vi "ATF-P&ID.vi"() -> ()   [LabVIEW 2022 SP3]
uses:
  Source code/Globals/Main_global.vi
  Source code/Globals/ATF1_NS_globals.vi
  <vilib>/Utility/error.llb/DialogType.ctl
  <vilib>/Waveform/DWDTOps.llb/DWDT Digital to Boolean Array.vi
  Source code/Globals/ATF1_ACQ.vi
  Source code/ATF_Queues/ATF_Message Cluster.ctl
  Source code/User Event - Stop/User Event - Stop.lvlib
  <vilib>/Analysis/3filter.llb/Filter Passband Type.ctl
  <vilib>/Analysis/NI_AALBase.lvlib
  <vilib>/ptbypt/NI_PtbyPt.lvlib
panel:
  out "Boolean 73":bool
  out "Boolean 30":bool
  in  "F EPV 1008":bool
  out "NC EPV 1008 HSS":bool
  out "Boolean 27":bool
  in  "F EPV 1007":bool
  out "F EPV 1007 HSS":bool
  in  "F EPV 1004":bool
  out "NC EPV 1004 HSS":bool
  out "Boolean 26":bool
  in  "NC EPV 1001":bool
  out "NC EPV 1001 HSS":bool
  out "Boolean 23":bool
  out "Boolean 25":bool
  out "NO EPV 477 HSS  3":bool
  in  "NC EPV 61":bool
  out "Boolean 104":bool
  out "Boolean 47":bool
  out "Boolean 3":bool
  out "Boolean 24":bool
  out "NC EPV 56 HSS":bool
  in  "NC EPV 56":bool
  out "Boolean 16":bool
  out "Boolean 116":bool
  in  "NO EPV 122":bool
  out "Boolean 46":bool
  out "NO EPV 1102 HSS 2":bool
  out "Boolean 103":bool
  out "F_RTD_56(K)":dbl format="%.2g"
  out "N_PT_121":dbl format="%.2g"
  out "WTT_LS 2":dbl(slide) scale=0.1..100.0
  out "Boolean 71":bool
  out "F_RTD_1013 (K)":dbl format="%.2g"
  out "PT SC":dbl format="%.2g"
  out "W_RTD_1177 (K)":dbl format="%.2g"
  out "F_SC_RTD(K)":dbl format="%.2g"
  out "PT 1000(K)":dbl format="%.2g"
  out "PT 1000-2 (K)":dbl format="%.2g"
  out "F_PT_1013b (bar)":dbl format="%.2g"
  out "F_PT_1013a (bar)":dbl format="%.2g"
  out "F_PT_1019":dbl format="%.2g"
  out "F_TCV_1018":dbl format="%.2g"
  out "TCV_1018(FB) %":dbl format="%.2g"
  out "Boolean 108":bool
  out "Boolean 107":bool
  out "F_RTD_1011(K)":dbl format="%.2g"
  out "Boolean 21":bool
  out "Boolean 138":bool
  out "Boolean 29":bool
  out "Boolean 28":bool
  out "F_PT_1011a (bar)":dbl format="%.2g"
  out "F_PT_1011b (bar)":dbl format="%.2g"
  out "F_FM_1010 (kg/s)":dbl format="%.2g"
  out "Boolean 106":bool
  out "Boolean 105":bool
  out "Boolean 121":bool
  out "Boolean 126":bool
  out "Boolean 109":bool
  out "Boolean 6":bool
  out "Boolean 81":bool
  out "NO EPV 477 HSS  2":bool
  in  "NO EPV 477":bool
  in  "NO EPV 478R":bool
  out "NO EPV 1207 HSS 2":bool
  out "Boolean 54":bool
  out "Boolean 53":bool
  out "Boolean 22":bool
  out "Boolean 86":bool
  out "F_PT_56 _R":dbl format="%.2g"
  in  "NC EPV 481":bool
  out "NC EPV 481 HSS":bool
  out "Boolean 85":bool
  out "F_PT_56":dbl format="%.2g"
  out "Boolean 115":bool
  out "Boolean 52":bool
  out "N_PT_480":dbl format="%.2g"
  out "Boolean 120":bool
  out "Boolean 72":bool
  out "Boolean 119":bool
  out "Boolean 13":bool
  out "N_PT_ATF_Cyl":dbl format="%.2g"
  out "Boolean 83":bool
  out "Boolean 102":bool
  out "Boolean 82":bool
  out "Boolean 101":bool
  out "N_PT_1101":dbl format="%.2g"
  out "N_PT_1090   2":dbl format="%.2g"
  in  "N EPV 1091":bool
  out "NO EPV 1091 HSS":bool
  out "Boolean 20":bool
  out "Boolean 118":bool
  in  "NC EPV 1217":bool
  out "NC EPV 1217 HSS":bool
  out "Boolean 4":bool
  out "Boolean 114":bool
  out "Boolean 12":bool
  out "N_PT_Water_Cyl":dbl format="%.2g"
  out "Boolean 79":bool
  out "N_PT_1210":dbl format="%.2g"
  out "Boolean 117":bool
  out "W_PT_1212":dbl format="%.2g"
  out "W_RTD_1212(K)":dbl format="%.2g"
  out "Boolean 19":bool
  out "Boolean 18":bool
  out "Boolean 8":bool
  out "Boolean 15":bool
  out "Boolean 14":bool
  out "Boolean 11":bool
  out "Boolean 10":bool
  in  "AC Button":bool
  in  "NO EPV 1207":bool
  out "Boolean 7":bool
  out "Boolean 5":bool
  in  "NC EPV 1214":bool
  out "Boolean 141":bool
  out "Boolean 9":bool
  out "WTT_LS":dbl(slide) scale=0.1..100.0
  out "Boolean 140":bool
  out "Boolean 144":bool
  out "Boolean 128":bool
  out "Boolean 125":bool
  in  "NO EPV 1102":bool
  out "Boolean 45":bool
  out "NC EPV 1211 HSS":bool
  in  "NC EPV 1211":bool
  out "NO EPV 1207 HSS":bool
  out "NC EPV 1214 HSS":bool
  out "NO EPV 1102 HSS":bool
  out "Boolean 113":bool
  out "Boolean 2":bool
  out "Boolean 100":bool
  out "Boolean 80":bool
  out "Boolean 78":bool
  out "Boolean 70":bool
  out "Boolean":bool
  out "Boolean 51":bool
  out "Boolean 17":bool
  out "Boolean 112":bool
  out "error out":errorcluster
  out "Sampling Rate_Accelerometer":dbl
  out "register values":u16[](array[numeric])
  # "ATF PUMP & STOORAGE P&ID"
  # "WTT\nh(mm)"
  # "ATF"
  # "ATF"
  # "ATF STORAGE\nAREA"
  # "ATF PUMP\nAREA"
  # "GN2"
  # "GN2"
  # "Version:V0.1"
  # "Release Date:14/10/2024"
  # "GN2"
  # "GN2"
  # "GN2"
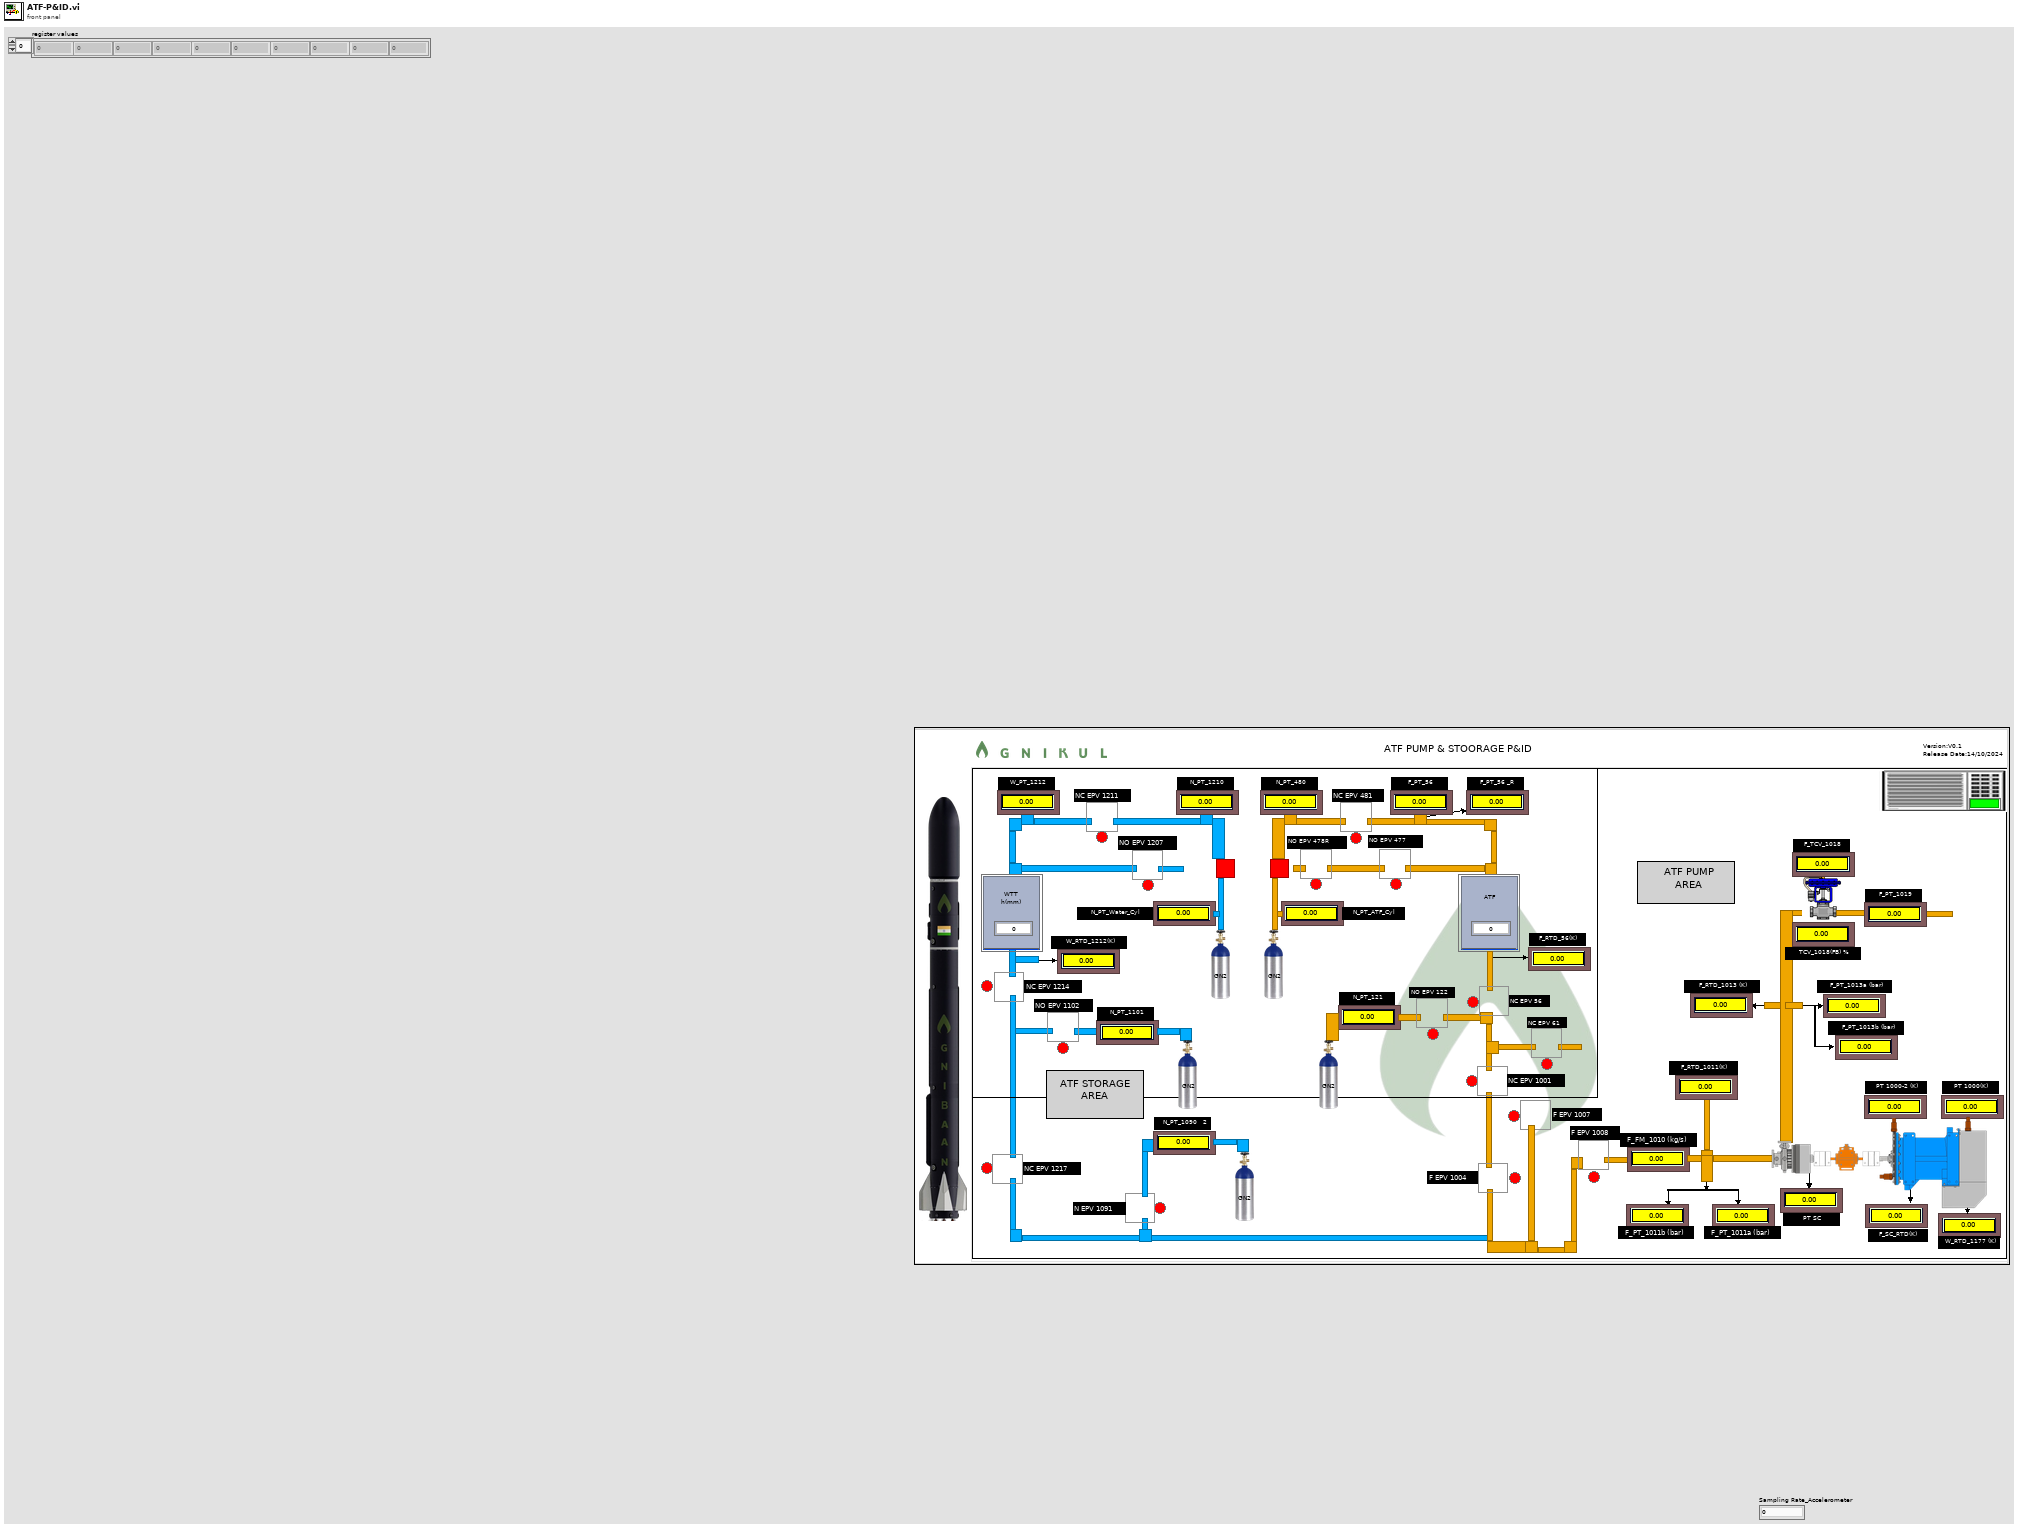
[diagram p1: front panel]
types:
  T1 = cluster{"DO Data":waveform(dbl)[], "DI Data":digitalwaveform[], "AI Data":waveform(dbl)[]}
  T2 = enum8{"Enabled", "Disabled", "Disabled and Grayed Out"}
  T3 = cluster{"UI":refnum<queue>, "Acquisition":refnum<queue>, "Logging":refnum<queue>}
  T4 = cluster{cluster{"AI":cluster{"AI signal Lists":string, "AI Channel List":string, "Prescale Min":dbl, "Prescale Max":dbl, "Prescale Unit":string, "Sensor Min":dbl, "Sensor Max":dbl, "Sensor Unit":string}[], "AI Sample rate":u32[], "AI Device list ":string[]}, cluster{"AO":cluster{"AO signal List":string, "AO Channel List":string, "AO Default Value":dbl}[], "AO Sample rate ":u32[], "AO Device list":string[]}, cluster{"DI":cluster{"DI Signal List":string, "DI Channel list":string, "Default":bool, "Inverted":bool}[], "DI Sample rate":u32[], "DI Device list  ":string[]}, cluster{"DO":cluster{"DO Signal List":string, "DO Channel List":string, "DO Default":bool, "DO Inverted":bool}[], "DO Sample rate":u32[], "DO Device list ":string[]}, cluster{"CI":cluster{"CI Signal list":string, "CI Channel List":string, "Initial Count":u32, "Count Direction":i32, "Edge":i32}[], "CI Sample rate":u32[], "CI Device list ":string[]}, cluster{"TC":cluster{"TC signal Lists":string, "TC Channel Lists":string, "TC type":i32, "Max.Value":dbl, "Min.Value":dbl, "Units":i32}[], "TC Sample rate":u32[], "TC Device list":string[]}, cluster{"Accelerometer":cluster{"name to assign":string, "physical channels":tag, "minimum value":dbl, "maximum value":dbl, "sensitivity":dbl, "sensitivity units":i32, "units":i32}[], "Acc Sampling Rate":string}}
  T5 = enum32{"Invalid", "Standard", "Closed", "Hidden", "Minimized", "Maximized"}
  T6 = typedef "Control 3.ctl" = cluster{"Info  Folder path":path, " Data Log Folder Path ":path, " Error log Folder Path":path, "Login Details  Folder Path":path, "HW Configaration  Folder Path":path, "Signal Folder Path":path, "Test Settings Data Log Folder Path ":path, "System Setting Sequence Folder Path":path, "Sequence Folder Path":path, "Sub VI's  Folder Path":path, "DAQ  VI's  Folder Path":path, "Source Code  Folder Path":path, "Log In Module  Folder Path ":path, "Button Operations Folder Path":path, "Loading Vi path":path, "Loading Vi path D":path}
  T7 = typedef "ATF_Message Cluster.ctl" = cluster{"Message":string, "Message Data":variant}
  T8 = typedef "DialogType.ctl" = u16
  T9 = typedef "NI_AALBase.lvlib/Filter Passband Type.ctl" = enum32{"Lowpass", "Highpass", "Bandpass", "Bandstop"}
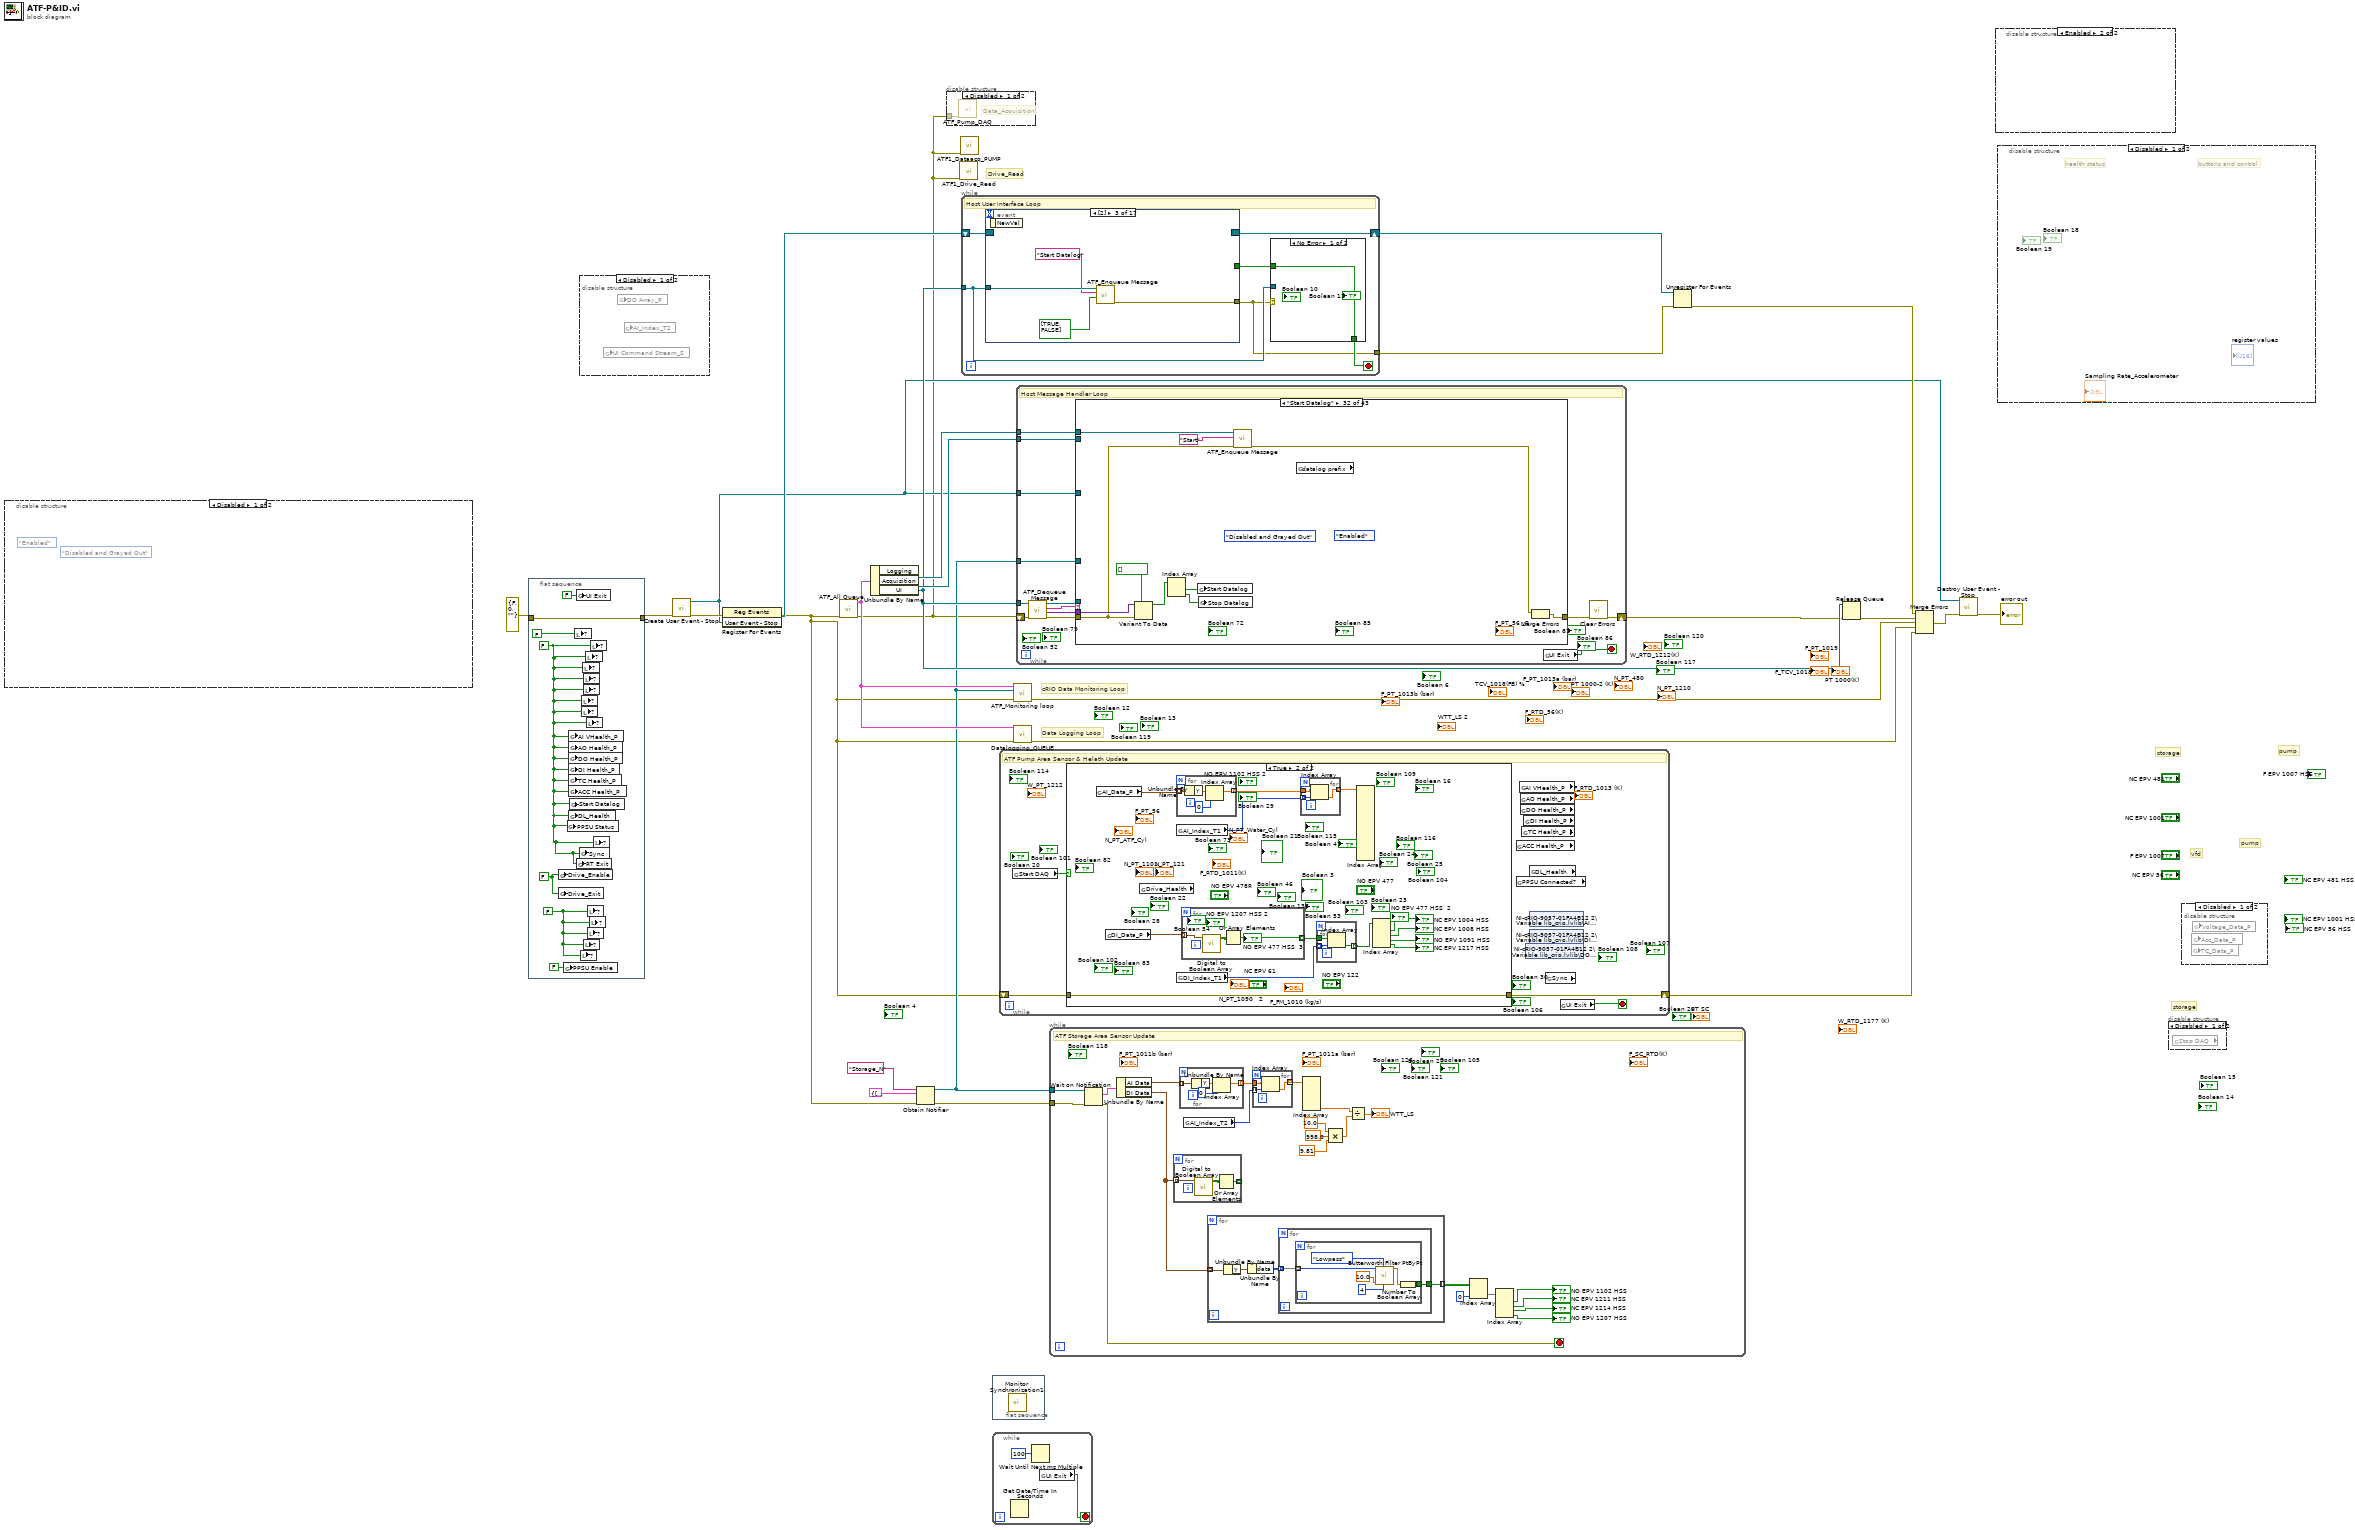
[diagram p0: block diagram]
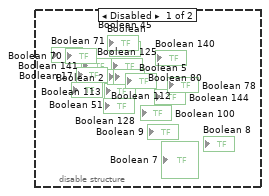
[diagram p7: hidden frame]
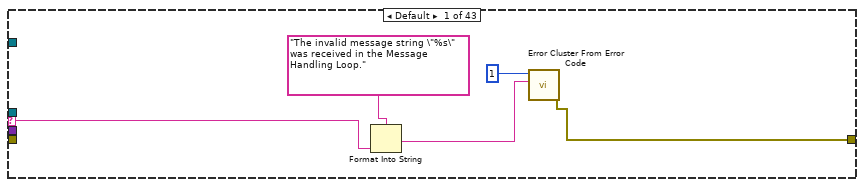
[diagram p9: hidden frame]
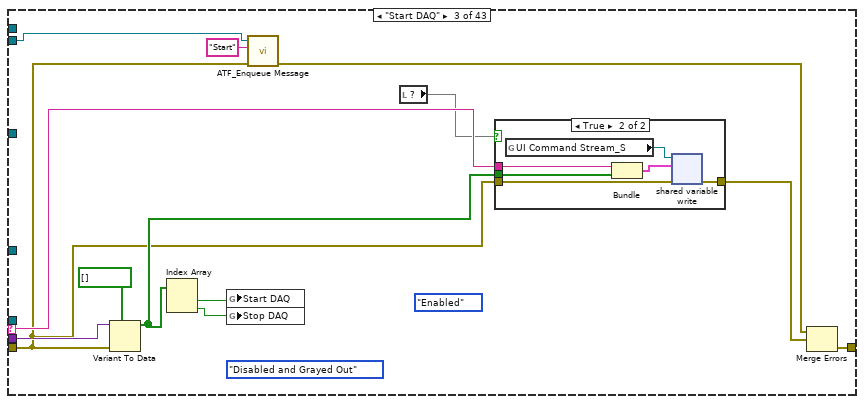
[diagram p11: hidden frame]
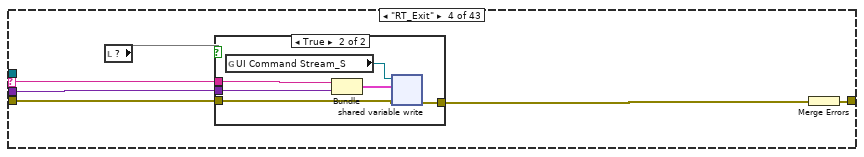
[diagram p13: hidden frame]
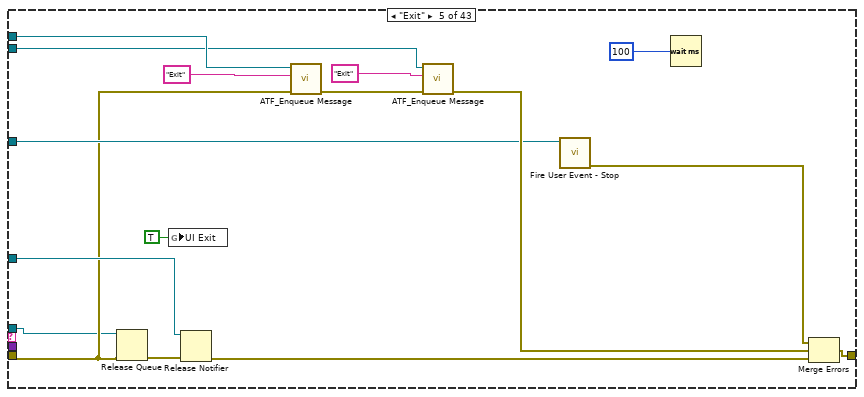
[diagram p15: hidden frame]
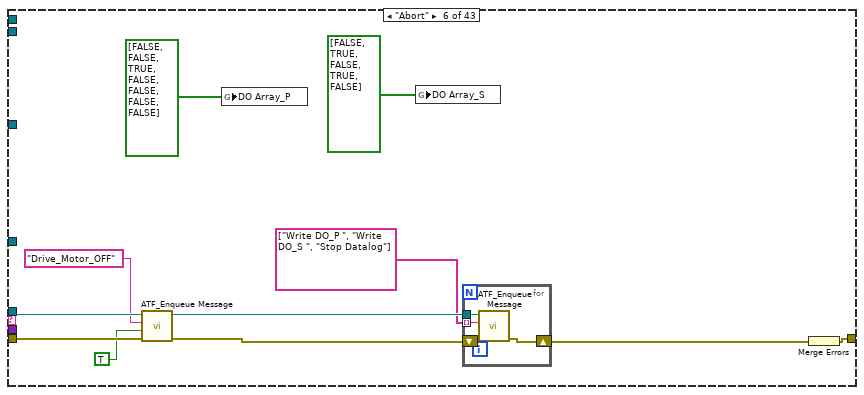
[diagram p16: hidden frame]
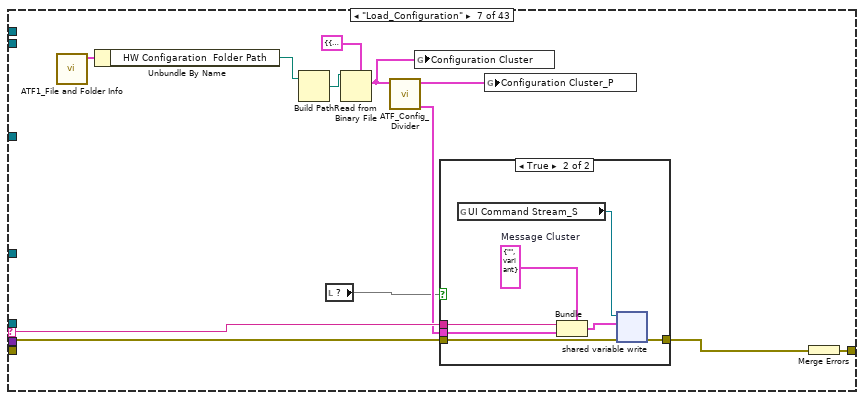
[diagram p17: hidden frame]
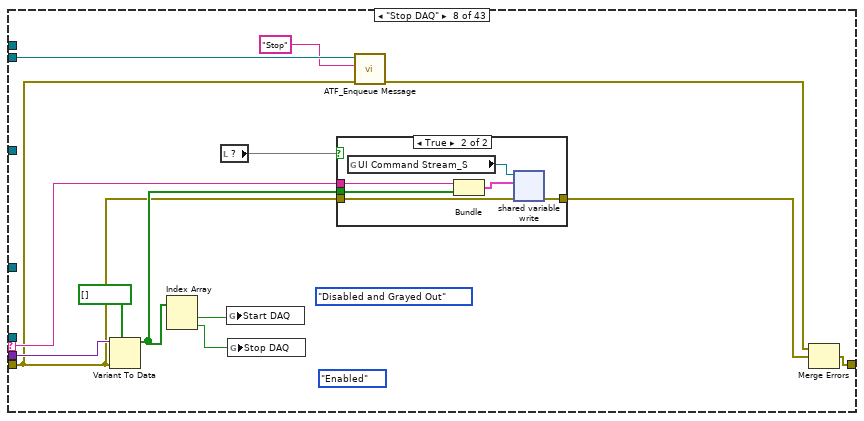
[diagram p19: hidden frame]
diagram:
  # "Data Logging Loop"
  # "cRIO Data Monitoring Loop"
  # "Drive_Read"
  # "pump"
  # "vfd"
  # "pump"
  # "storage"
  # "storage"
  n1 = disable-structure shown="Disabled" {
    frame Disabled {
      w27 = T2."Disabled and Grayed Out" ("Disabled")
      w26 = T2."Enabled" ("Disabled")
    }
    frame Enabled {
    }
  }
  n2 = flat-sequence {
    tunnel: [w29] -> w4
    tunnel: errorcluster {"status"=FALSE, "code"=0, "source"=""} ("error in (no error)") -> [w29]
    frame #0 {
      w31 = FALSE ("DI Health cRIO")
      w32 = FALSE ("Drive Connected?")
      w28 = FALSE ("Datalog Health")
      n3 = global write "ATF1_ACQ.vi" "Drive_Enable"(w32) -> ()
      n4 = global write "ATF1_ACQ.vi" "Drive_Exit"(w32) -> ()
      n5 = global write "Main_global.vi" "PPSU Enable"(FALSE ("PPSU Enable")) -> ()
      n6 = global write "ATF1_ACQ.vi" "PPSU Status"(w28) -> ()
      n7 = global write "ATF1_ACQ.vi" "AI VHealth_P"(w28) -> ()
      n8 = global write "ATF1_ACQ.vi" "AO Health_P"(w28) -> ()
      n9 = global write "ATF1_ACQ.vi" "DO Health_P"(w28) -> ()
      n10 = global write "ATF1_ACQ.vi" "DI Health_P"(w28) -> ()
      n11 = global write "ATF1_ACQ.vi" "TC Health_P"(w28) -> ()
      n12 = global write "ATF1_ACQ.vi" "ACC Health_P"(w28) -> ()
      n13 = global write "Main_global.vi" "DL_Health"(w28) -> ()
      n14 = global write "Main_global.vi" "Start Datalog"(w28) -> ()
      n15 = local write item#-1(FALSE ("PUMP Connected?")) -> ()
      n16 = global write "Main_global.vi" "UI Exit"(FALSE ("UI Exit")) -> ()
      n17 = global write "Main_global.vi" "RT Exit"(w28) -> ()
      n18 = global write "Main_global.vi" "Sync"(w28) -> ()
      n19 = local write item#-1(w31) -> ()
      n20 = local write item#-1(w28) -> ()
      n21 = local write item#-1(w28) -> ()
      n22 = local write item#-1(w28) -> ()
      n23 = local write item#-1(w28) -> ()
      n24 = local write item#-1(w28) -> ()
      n25 = local write item#-1(w31) -> ()
      n26 = local write item#-1(w28) -> ()
      n27 = local write item#-1(w28) -> ()
      n28 = local write item#-1(w31) -> ()
      n29 = local write item#-1(w31) -> ()
      n30 = local write item#-1(w31) -> ()
      n31 = local write item#-1(w28) -> ()
      n32 = local write item#-1(w28) -> ()
    }
  }
  n33 = disable-structure shown="Disabled" {
    frame Disabled {
      n34 = global read "ATF1_NS_globals.vi" "UI Command Stream_S"() -> ()  [unwired: 1 in]
      n35 = global read "ATF1_ACQ.vi" "DO Array_P"() -> ()  [unwired: 1 in]
      n36 = global read "Main_global.vi" "AI_Index_T2"() -> ()  [unwired: 1 in]
    }
    frame Enabled {
    }
  }
  n37 = call "Create User Event - Stop.vi"("error in (no error)"=w4) -> ("error out"=w13:errorcluster, "User Event - Stop"=w6:refnum<user-event>)  [unwired: 9 in]
  n38 = register-events(error in=w13, w6) -> (reference out=w12:refnum<event-registration>, error out=w2:errorcluster)  [unwired: 1 in]
  n39 = call "ATF_All Queue.vi"("error in"=w2) -> ("error out"=w1:errorcluster, "Cluster"=w19:T3)  [unwired: 9 in]
  n40 = Unbundle By Name(w19) -> ("Logging"=w25:refnum<queue>, "Acquisition"=w24:refnum<queue>, "UI"=w23:refnum<queue>)
  n41 = Obtain Notifier(name (unnamed)="Storage_N", notification data type=T1 {"DO Data"=[], "DI Data"=[], "AI Data"=[]}, error in (no error)=w2) -> (notifier out=w14:refnum<notifier>, error out=w16:errorcluster)  [unwired: 1 in, 1 out]
  n42 = disable-structure shown="Disabled" {
    disable-tunnel: w1 -> [w35 _]
    frame Disabled {
      # "Data_Acquisition"
      n43 = call "ATF_Pump_DAQ.vi"("error constant"=w35) -> ()  [unwired: 10 in, 1 out]
    }
    frame Enabled {
    }
  }
  n44 = call "ATF1_Drive_Read.vi"("error in (no error)"=w1) -> ()  [unwired: 10 in, 1 out]
  n45 = call "ATF1_Dataacq_PUMP.vi"("error In"=w1) -> ()  [unwired: 10 in, 1 out]
  n46 = while {
    tunnel: w23 -> [w41]
    shift-right: [w37] -> w10
    shift-left: w12 -> [w38]
    tunnel: [w36] -> w11
    stop <- w40 stop-if-true
    # "Host User Interface Loop"
    n47 = event shown="[2]" {
      selector: w38 -> [_ _ _ _ _ _ _ _ _ _ _ _ _ _ _ _ _]
      dyn-events: [_ _ _ _ _ _ _ _ _ _ _ _ _ _ _ _ _] -> w37
      timeout: _ -> [_ _ _ _ _ _ _ _ _ _ _ _ _ _ _ _ _]
      tunnel: w41 -> [w49 w61 w65 w68 w72 w77 w82 w86 w90 w94 w97 w101 w105 w108 w111 _ w118]
      tunnel: [w53 w60 w64 w67 w71 w76 w81 w85 w89 w93 w96 w100 w104 w107 w110 _ w116] -> w36
      tunnel: [_ _ _ _ _ TRUE _ _ _ _ _ _ _ _ _ TRUE ("Discard?") _] -> w39
      event #0 (no event record) {
        n48 = event-data() -> ()  [unwired: 1 in, 1 out]
        n49 = for {
          tunnel: [w57] -> w50
          tunnel: w49 -> [w56]
          tunnel: [w55] -> w48
          tunnel: string[] ["Load_Configuration", "Signal_List", "Indexing", "Update DO_P", "Update DO_S", "Write DO_P", "Write DO_S"] -> [w54] mode=indexing
          n50 = call "ATF_Enqueue Message.vi"("Message"=w54, "Message Queue"=w56) -> ("error out"=w57:errorcluster, "dup Message Queue"=w55:refnum<queue>)  [unwired: 8 in]
        }
        n51 = call "ATF_Enqueue Message.vi"("error in (no error)"=w50, "Message Data"=bool[] [TRUE, FALSE], "Message"="Start DAQ", "Message Queue"=w48) -> ("error out"=w53:errorcluster)  [unwired: 6 in, 1 out]
      }
      event #1 (no event record) {
        n52 = event-data() -> ()  [unwired: 1 in, 1 out]
        n53 = call "ATF_Enqueue Message.vi"("Message Data"=bool[] [FALSE, TRUE], "Message"="Stop DAQ", "Message Queue"=w61) -> ("error out"=w60:errorcluster)  [unwired: 7 in, 1 out]
      }
      event #2 (no event record) {
        n54 = event-data() -> ()  [unwired: 1 in, 1 out]
        n55 = call "ATF_Enqueue Message.vi"("Message Data"=bool[] [TRUE, FALSE], "Message"="Start Datalog", "Message Queue"=w65) -> ("error out"=w64:errorcluster)  [unwired: 7 in, 1 out]
      }
      event #3 (no event record) {
        n56 = event-data() -> ()  [unwired: 1 in, 1 out]
        n57 = call "ATF_Enqueue Message.vi"("Message"="Rename_Datalog", "Message Queue"=w68) -> ("error out"=w67:errorcluster)  [unwired: 8 in, 1 out]
      }
      event #4 (no event record) {
        n58 = event-data() -> ()  [unwired: 1 in, 1 out]
        n59 = call "ATF_Enqueue Message.vi"("Message Data"=bool[] [FALSE, TRUE], "Message"="Stop Datalog", "Message Queue"=w72) -> ("error out"=w71:errorcluster)  [unwired: 7 in, 1 out]
      }
      event #5 (no event record) {
        n60 = event-data() -> ()  [unwired: 1 in, 1 out]
        n61 = call "ATF_Enqueue Message.vi"("Message"="Exit", "Message Queue"=w77) -> ("error out"=w76:errorcluster, "Message Data"=w73:variant)  [unwired: 7 in, 1 out]
      }
      event #6 (no event record) {
        n62 = event-data() -> ("NewVal"=w79)  [unwired: 1 in]
        n63 = call "ATF_Enqueue Message.vi"("Message Data"=w79, "Message"="RT_Exit", "Message Queue"=w82) -> ("error out"=w81:errorcluster)  [unwired: 7 in, 1 out]
        n64 = global read "Main_global.vi" "RT Exit"() -> (w78:bool)
      }
      event #7 (no event record) {
        n65 = event-data() -> ("NewVal"=w83)  [unwired: 1 in]
        n66 = call "ATF_Enqueue Message.vi"("Message Data"=w83, "Message"="DAQ_Configuration", "Message Queue"=w86) -> ("error out"=w85:errorcluster)  [unwired: 7 in, 1 out]
      }
      event #8 (no event record) {
        n67 = event-data() -> ("NewVal"=w87)  [unwired: 1 in]
        n68 = call "ATF_Enqueue Message.vi"("Message Data"=w87, "Message"="VFD Settings", "Message Queue"=w90) -> ("error out"=w89:errorcluster)  [unwired: 7 in, 1 out]
      }
      event #9 (no event record) {
        n69 = event-data() -> ("NewVal"=w91)  [unwired: 1 in]
        n70 = call "ATF_Enqueue Message.vi"("Message Data"=w91, "Message"="RT Connect", "Message Queue"=w94) -> ("error out"=w93:errorcluster)  [unwired: 7 in, 1 out]
      }
      event #10 (no event record) {
        n71 = event-data() -> ()  [unwired: 1 in, 3 out]
        n72 = call "ATF_Enqueue Message.vi"("Message"="Update_HW_File_List", "Message Queue"=w97) -> ("error out"=w96:errorcluster)  [unwired: 8 in, 1 out]
      }
      event #11 (no event record) {
        n73 = event-data() -> ()  [unwired: 1 in, 1 out]
        n74 = call "ATF_Enqueue Message.vi"("Message"="Abort", "Message Queue"=w101) -> ("error out"=w100:errorcluster, "Message Data"=w98:variant)  [unwired: 7 in, 1 out]
      }
      event #12 (no event record) {
        n75 = event-data() -> ("NewVal"=w102)  [unwired: 1 in]
        n76 = call "ATF_Enqueue Message.vi"("Message Data"=w102, "Message"="Edit IP", "Message Queue"=w105) -> ("error out"=w104:errorcluster)  [unwired: 7 in, 1 out]
      }
      event "F EPV 1004", "F EPV 1008", "N EPV 1091", "NC EPV 1217": Value Change {
        n77 = event-data() -> ()  [unwired: 1 in, 1 out]
        n78 = call "ATF_Enqueue Message.vi"("Message"="Write DO_P", "Message Queue"=w108) -> ("error out"=w107:errorcluster)  [unwired: 8 in, 1 out]
      }
      event "NC EPV 1214", "NO EPV 1102", "NO EPV 1207", "NC EPV 1211", "AC Button": Value Change {
        n79 = event-data() -> ()  [unwired: 1 in, 1 out]
        n80 = call "ATF_Enqueue Message.vi"("Message"="Write DO_S", "Message Queue"=w111) -> ("error out"=w110:errorcluster)  [unwired: 8 in, 1 out]
      }
      event User Event {
        n81 = event-data() -> ()  [unwired: 1 in, 3 out]
      }
      event #16 (no event record) {
        n82 = event-data() -> ()  [unwired: 1 in, 3 out]
        n83 = Divide(y=10.0) -> (x=w115:dbl, x/y=w113:dbl)
        n84 = call "ATF_Enqueue Message.vi"("Message Data"=w113, "Message"="Control_Valve", "Message Queue"=w118) -> ("error out"=w116:errorcluster)  [unwired: 7 in, 1 out]
      }
    }
    n85 = case shown="No Error" w36 {
      tunnel: w41 -> [_ w46]
      tunnel: [w42 TRUE ("Priority Message? (F)")] -> w40
      tunnel: w39 -> [w42 _]
      frame No Error {
      }
      frame Error {
        n86 = call "ATF_Enqueue Message.vi"("Priority Message?"=TRUE ("Priority Message? (F)"), "Message"="Exit", "Message Queue"=w46) -> ()  [unwired: 7 in, 2 out]
      }
    }
  }
  n87 = while {
    stop <- w119 stop-if-true
    n88 = Get Date/Time In Seconds() -> (seconds since 1Jan1904=w121:timestamp)
    n89 = Wait Until Next ms Multiple(millisecond multiple=u32 100) -> ()  [unwired: 1 out]
    n90 = global read "Main_global.vi" "UI Exit"() -> (w119:bool)
  }
  n91 = flat-sequence {
    frame #0 {
      n92 = call "Monitor Synchronization1.vi"() -> ()  [unwired: 12 in]
    }
  }
  n93 = while {
    shift-right: [w132] -> w5
    shift-left: w2 -> [w133]
    stop <- w134 stop-if-true
    # "ATF Pump Area Sensor & Helath Update"
    n94 = global read "Main_global.vi" "Start DAQ"() -> (w135:bool)
    n95 = case shown="True" w135 {
      tunnel: w133 -> [w136 w138]
      tunnel: [w136 w138] -> w132
      frame False {
      }
      frame True {
        n96 = global read "ATF1_ACQ.vi" "AI_Data_P"() -> (w141:waveform(dbl)[])
        n97 = global read "ATF1_ACQ.vi" "DI_Data_P"() -> (w140:digitalwaveform[])
        n98 = global read "ATF1_ACQ.vi" "Drive_Health"() -> (w139:bool)
        n99 = for {
          tunnel: w141 -> [w177] mode=indexing
          tunnel: [w175] -> w144 mode=indexing
          n100 = Unbundle By Name(w177) -> ("Y"=w176:dbl[])
          n101 = Index Array(array=w176, index=0) -> (element=w175:dbl)
        }
        n102 = global read "Main_global.vi" "AI_Index_T1"() -> (w142:i32[])
        n103 = global read "Main_global.vi" "DI_Index_T1"() -> (w145:i32[])
        n104 = for {
          tunnel: [w172] -> w146 mode=indexing
          tunnel: w140 -> [w171] mode=indexing
          n105 = call-poly <vilib>:"Digital to Boolean Array.vi"("digital waveform"=w171) -> ("boolean array"=w173:bool[][])  [unwired: 9 in, 1 out]
          n106 = Or Array Elements(Boolean array=w173) -> (logical OR=w172:bool)
        }
        n107 = for {
          tunnel: w144 -> [w167]
          tunnel: [w166] -> w143 mode=indexing
          tunnel: w142 -> [w165] mode=indexing
          n108 = Index Array(array=w167, index=w165) -> (element=w166:dbl)
        }
        n109 = for {
          tunnel: w146 -> [w170]
          tunnel: [w169] -> w147 mode=indexing
          tunnel: w145 -> [w168] mode=indexing
          n110 = Index Array(array=w170, index=w168) -> (element=w169:bool)
        }
        n111 = Index Array(array=w143) -> (element #1=w164:dbl, element #2=w163:dbl, element #3=w162:dbl, element #4=w161:dbl, element #5=w160:dbl, element #6=w159:dbl, element #7=w137:dbl, element #8=w158:dbl, element #9=w157:dbl, element #10=w156:dbl, element #11=w155:dbl, element #12=w154:dbl, element #13=w153:dbl, element #14=w152:dbl)  [unwired: 14 in]
        n112 = Index Array(array=w147) -> (element #1=→"NC EPV 1004 HSS":bool, element #2=→"NC EPV 1008 HSS":bool, element #3=→"NO EPV 1091 HSS":bool, element #4=→"NC EPV 1217 HSS":bool)  [unwired: 4 in]
      }
    }
    n113 = global read "ATF1_ACQ.vi" "ACC Health_P"() -> (w131:bool)
    n114 = global read "ATF1_ACQ.vi" "PPSU Connected?"() -> (w124:bool)
    n115 = global read "ATF1_ACQ.vi" "AI VHealth_P"() -> (w130:bool)
    n116 = global read "ATF1_ACQ.vi" "AO Health_P"() -> (w129:bool)
    n117 = global read "ATF1_ACQ.vi" "DO Health_P"() -> (w128:bool)
    n118 = global read "ATF1_ACQ.vi" "TC Health_P"() -> (w126:bool)
    n119 = global read "ATF1_ACQ.vi" "DI Health_P"() -> (w127:bool)
    n120 = shared-variable "NI-cRIO-9057-01FA4B12 2\\Variable lib_crio.lvlib\\DO Health"() -> ()  [unwired: 1 in, 2 out]
    n121 = global read "Main_global.vi" "DL_Health"() -> (w125:bool)
    n122 = shared-variable "NI-cRIO-9057-01FA4B12 2\\Variable lib_crio.lvlib\\AI Health"() -> (w122:bool)  [unwired: 1 in, 1 out]
    n123 = shared-variable "NI-cRIO-9057-01FA4B12 2\\Variable lib_crio.lvlib\\DI Health"() -> ()  [unwired: 1 in, 2 out]
    n124 = global read "Main_global.vi" "Sync"() -> (w123:bool)
    n125 = global read "Main_global.vi" "UI Exit"() -> (w134:bool)
  }
  n126 = call "Datalogging_QUEUE.vi"("error in"=w2, "Message Queues"=w19) -> ("error out"=w18:errorcluster)  [unwired: 9 in]
  n127 = call "ATF_Monitoring loop.vi"("error in"=w2, "notifier"=w14, "Message Queues"=w19) -> ("error out"=w20:errorcluster)  [unwired: 8 in]
  n128 = while {
    tunnel: w23 -> [w181]
    shift-right: [w189] -> w22
    shift-left: w1 -> [w182]
    tunnel: w25 -> [w187]
    tunnel: w24 -> [w186]
    tunnel: w14 -> [w185]
    tunnel: w6 -> [w184]
    stop <- w188 stop-if-true
    # "Host Message Handler Loop"
    n129 = call "ATF_Dequeue Message.vi"("Message Queue"=w181, "error IO"=w182) -> ("dup Message Queus"=w180:refnum<queue>, "Message"=w178:string, "Message Data"=w179:variant, "error out"=w183:errorcluster)  [unwired: 4 in]
    n130 = case shown="\"Start Datalog\"" w178 {
      selector: w178 -> [w192 _ w209 w226 _ _ w277 w298 _ _ _ _ _ _ _ _ _ _ _ _ _ _ _ _ _ _ _ _ _ _ _ _ _ _ _ _ _ _ _ _ w585 _ _]
      tunnel: w180 -> [_ _ _ _ w235 w258 _ _ _ _ _ _ _ _ _ _ _ _ _ _ _ _ _ _ _ _ _ _ _ _ _ _ _ _ w524 _ _ _ _ _ _ _ _]
      tunnel: w179 -> [_ _ w213 w222 _ _ _ w302 w314 w317 _ _ _ _ _ _ w339 _ _ _ w370 w386 w400 w415 _ _ w446 _ _ w464 _ w486 _ w517 _ _ _ _ _ _ _ _ _]
      tunnel: w183 -> [_ w196 w197 w221 w237 w259 w274 w288 w313 w320 w322 w324 w326 w330 w332 w335 w342 w345 w348 w353 w371 w387 w402 w416 w429 w439 w449 w454 w461 w466 w470 w476 w489 w508 w523 w531 _ _ _ w577 w587 w596 _]
      tunnel: [w191 w196 w206 w224 w249 w260 w276 w295 w315 w321 w323 w325 w327 w331 w334 w337 w343 w346 w349 w352 w373 w388 w403 w418 w430 w443 w448 w459 w462 w469 w471 w475 w492 w506 w527 w531 _ _ _ w576 w586 w597 _] -> w190
      tunnel: w187 -> [_ _ _ _ w246 _ _ _ _ _ _ _ _ _ _ _ _ _ _ _ _ _ _ _ _ _ _ _ _ _ _ w477 w488 w507 _ _ _ _ _ _ _ _ _]
      tunnel: w186 -> [_ _ w200 _ w244 _ _ w289 _ _ _ _ _ _ _ _ _ _ _ _ _ _ _ _ _ _ _ _ _ _ _ _ _ _ _ _ _ _ _ _ _ _ _]
      tunnel: w185 -> [_ _ _ _ w247 _ _ _ _ _ _ _ _ _ _ _ _ _ _ _ _ _ _ _ _ _ _ _ _ _ _ _ _ _ _ _ _ _ _ _ _ _ _]
      tunnel: w184 -> [_ _ _ _ w238 _ _ _ _ _ _ _ _ _ _ _ _ _ _ _ _ _ _ _ _ _ _ _ _ _ _ _ _ _ _ _ _ _ _ _ _ _ _]
      frame Default {
        n131 = Format Into String(format string="The invalid message string \"%s\" was received in the Message Handling Loop." ("Invalid Message Loop Message"), w192) -> (resulting string=w193:string)  [unwired: 2 in, 1 out]
        n132 = call <vilib>:"Error Cluster From Error Code.vi"("error message (\"\")"=w193, "error code (0)"=1) -> ("error out"=w191:errorcluster)  [unwired: 7 in]
      }
      frame "Initialize" {
      }
      frame "Start DAQ" {
        w201 = T2."Enabled" ("Disabled")
        w204 = T2."Disabled and Grayed Out" ("Disabled")
        n133 = Variant To Data(error in=w197, type=bool[] [], Variant=w213) -> (data=w208:bool[], error out=w203:errorcluster)
        n134 = Index Array(array=w208) -> (element #1=w211:bool, element #2=w210:bool)  [unwired: 2 in]
        n135 = global write "Main_global.vi" "Start DAQ"(w211) -> ()
        n136 = global write "Main_global.vi" "Stop DAQ"(w210) -> ()
        n137 = call "ATF_Enqueue Message.vi"("error in (no error)"=w197, "Message"="Start", "Message Queue"=w200) -> ("error out"=w198:errorcluster)  [unwired: 7 in, 1 out]
        n138 = local read item#-1() -> (w207)
        n139 = case shown="True" w207 {
          tunnel: [w214 w220] -> w205
          tunnel: w209 -> [_ w219]
          tunnel: w208 -> [_ w216]
          tunnel: w197 -> [w214 w215]
          frame False {
          }
          frame True {
            n140 = global read "ATF1_NS_globals.vi" "UI Command Stream_S"() -> (w217:refnum<k21>)
            n141 = Bundle(w219, w216) -> (w218:cluster{string, bool[]})  [unwired: 1 in]
            n142 = shared-variable-write(w217, w215, w218) -> (w220:errorcluster)  [unwired: 1 in, 2 out]
          }
        }
        n143 = Merge Errors(w198, w205) -> (w206:errorcluster, w202:errorcluster)
      }
      frame "RT_Exit" {
        n144 = local read item#-1() -> (w225)
        n145 = case shown="True" w225 {
          tunnel: [w227 w233] -> w223
          tunnel: w226 -> [_ w232]
          tunnel: w222 -> [_ w229]
          tunnel: w221 -> [w227 w228]
          frame False {
          }
          frame True {
            n146 = global read "ATF1_NS_globals.vi" "UI Command Stream_S"() -> (w230:refnum<k21>)
            n147 = Bundle(w232, "Message Data"=w229) -> (w231:cluster{string, "Message Data":variant})  [unwired: 1 in]
            n148 = shared-variable-write(w230, w228, w231) -> (w233:errorcluster)  [unwired: 1 in, 2 out]
          }
        }
        n149 = Merge Errors(w223) -> (w224:errorcluster)
      }
      frame "Exit" {
        n150 = Release Queue(queue=w235, error in (no error)=w237) -> (error out=w236:errorcluster)  [unwired: 1 in, 2 out]
        n151 = global write "Main_global.vi" "UI Exit"(TRUE ("UI Exit")) -> ()
        n152 = Release Notifier(notifier=w247, error in (no error)=w236) -> (error out=w245:errorcluster)  [unwired: 1 in, 2 out]
        n153 = call "ATF_Enqueue Message.vi"("error in (no error)"=w237, "Message"="Exit", "Message Queue"=w246) -> ("error out"=w240:errorcluster)  [unwired: 7 in, 1 out]
        n154 = call "ATF_Enqueue Message.vi"("error in (no error)"=w240, "Message"="Exit", "Message Queue"=w244) -> ("error out"=w241:errorcluster)  [unwired: 7 in, 1 out]
        n155 = call "Fire User Event - Stop.vi"("User Event - Stop"=w238) -> ("error out"=w239:errorcluster)  [unwired: 10 in]
        n156 = Wait (ms)(milliseconds to wait=u32 100) -> ()  [unwired: 1 out]
        n157 = Merge Errors(w239, w241, w245) -> (w249:errorcluster)
      }
      frame "Abort" {
        n158 = call "ATF_Enqueue Message.vi"("error in (no error)"=w259, "Message Data"=TRUE, "Message"="Drive_Motor_OFF", "Message Queue"=w258) -> ("error out"=w255:errorcluster, "dup Message Queue"=w253:refnum<queue>)  [unwired: 6 in]
        n159 = global write "ATF1_ACQ.vi" "DO Array_P"(bool[] [FALSE, FALSE, TRUE, FALSE, FALSE, FALSE, FALSE] ("DO Array_P")) -> ()
        n160 = global write "ATF1_ACQ.vi" "DO Array_S"(bool[] [FALSE, TRUE, FALSE, TRUE, FALSE] ("DO Array_S")) -> ()
        n161 = for {
          tunnel: w253 -> [w262]
          tunnel: string[] ["Write DO_P ", "Write DO_S ", "Stop Datalog"] -> [w261] mode=indexing
          shift-right: [w263] -> w254
          shift-left: w255 -> [w264]
          n162 = call "ATF_Enqueue Message.vi"("error in (no error)"=w264, "Message"=w261, "Message Queue"=w262) -> ("error out"=w263:errorcluster)  [unwired: 7 in, 1 out]
        }
        n163 = Merge Errors(w254) -> (w260:errorcluster)
      }
      frame "Load_Configuration" {
        n164 = call "ATF1_File and Folder Info.vi"() -> ("Path Cluster 3"=w270:T6)  [unwired: 10 in, 1 out]
        n165 = Unbundle By Name(w270) -> ("HW Configaration  Folder Path"=w271:path)
        n166 = Build Path(base path=w271) -> (name or relative path=w272:path, appended path=w273:path)
        n167 = local read item#-1() -> (w266)
        n168 = Read from Binary File(5:T4 {{"AI"=[], "AI Sample rate"=[], "AI Device list "=[]}, {"AO"=[], "AO Sample rate "=[], "AO Device list"=[]}, {"DI"=[], "DI Sample rate"=[], "DI Device list  "=[]}, {"DO"=[], "DO Sample rate"=[], "DO Device list "=[]}, {"CI"=[], "CI Sample rate"=[], "CI Device list "=[]}, {"TC"=[], "TC Sample rate"=[], "TC Device list"=[]}, {"Accelerometer"=[], "Acc Sampling Rate"=""}} ("Configuration Cluster"), 11:w273) -> (2:w267:T4)  [unwired: 4 in, 3 out]
        n169 = call "ATF_Config_Divider.vi"("Configuration Cluster"=w267) -> ("Configuration Cluster_S"=w269:T4, "Configuration Cluster_P"=w265:T4)  [unwired: 9 in]
        n170 = global write "Main_global.vi" "Configuration Cluster"(w267) -> ()
        n171 = case shown="True" w266 {
          tunnel: [w278 w285] -> w275
          tunnel: w277 -> [_ w284]
          tunnel: w274 -> [w278 w281]
          tunnel: w269 -> [_ w280]
          frame False {
          }
          frame True {
            w279 = T7 {"Message"="", "Message Data"=variant}  # Message Cluster
            n172 = global read "ATF1_NS_globals.vi" "UI Command Stream_S"() -> (w282:refnum<k21>)
            n173 = Bundle(cluster=w279, "Message"=w284, "Message Data"=w280) -> (w283:T7)
            n174 = shared-variable-write(w282, w281, w283) -> (w285:errorcluster)  [unwired: 1 in, 2 out]
          }
        }
        n175 = global write "Main_global.vi" "Configuration Cluster_P"(w265) -> ()
        n176 = Merge Errors(w275) -> (w276:errorcluster)
      }
      frame "Stop DAQ" {
        w290 = T2."Disabled and Grayed Out" ("Disabled")
        w293 = T2."Enabled" ("Disabled")
        n177 = Variant To Data(error in=w288, type=bool[] [], Variant=w302) -> (data=w297:bool[], error out=w292:errorcluster)
        n178 = Index Array(array=w297) -> (element #1=w300:bool, element #2=w299:bool)  [unwired: 2 in]
        n179 = local read item#-1() -> (w296)
        n180 = global write "Main_global.vi" "Start DAQ"(w300) -> ()
        n181 = global write "Main_global.vi" "Stop DAQ"(w299) -> ()
        n182 = case shown="True" w296 {
          tunnel: [w303 w309] -> w294
          tunnel: w298 -> [_ w308]
          tunnel: w297 -> [_ w305]
          tunnel: w288 -> [w303 w304]
          frame False {
          }
          frame True {
            n183 = global read "ATF1_NS_globals.vi" "UI Command Stream_S"() -> (w306:refnum<k21>)
            n184 = Bundle(w308, w305) -> (w307:cluster{string, bool[]})  [unwired: 1 in]
            n185 = shared-variable-write(w306, w304, w307) -> (w309:errorcluster)  [unwired: 1 in, 2 out]
          }
        }
        n186 = call "ATF_Enqueue Message.vi"("error in (no error)"=w288, "Message"="Stop", "Message Queue"=w289) -> ("error out"=w286:errorcluster)  [unwired: 7 in, 1 out]
        n187 = Merge Errors(w286, w294) -> (w295:errorcluster, w291:errorcluster)
      }
      frame "Set_RPM" {
        n188 = Variant To Data(error in=w313, type=0.0 ("Set RPM"), Variant=w314) -> (data=w310:dbl, error out=w312:errorcluster)
        n189 = global write "ATF1_ACQ.vi" "VFD_set_rpm"(w310) -> ()
        n190 = Merge Errors(w312) -> (w315:errorcluster)
      }
      frame "VFD_ON" {
        n191 = Variant To Data(error in=w320, type=0.0, Variant=w317) -> (data=w316:dbl, error out=w319:errorcluster)
        n192 = global write "ATF1_ACQ.vi" "VFD_ON"(w316) -> ()
        n193 = Merge Errors(w319) -> (w321:errorcluster)
      }
      frame "VFD_Enable" {
        n194 = Merge Errors(w322) -> (w323:errorcluster)
      }
      frame "VFD_Configuration" {
        n195 = Merge Errors(w324) -> (w325:errorcluster)
      }
      frame "PPSU_Update_Settings" {
        n196 = flat-sequence {
          frame #0 {
            n197 = call "ATF_PPSU control2.vi"() -> ()  [unwired: 27 in, 1 out]
          }
          frame #1 {
            n198 = One Button Dialog(message="PPSU Settings_Updated") -> ()  [unwired: 1 in, 1 out]
          }
        }
        n199 = Merge Errors(w326) -> (w327:errorcluster)
      }
      frame "PPSU Exit" {
        n200 = global write "ATF1_ACQ.vi" "PPSU Connected?"(FALSE ("PPSU Connected?")) -> ()
        n201 = Merge Errors(w330) -> (w331:errorcluster)
      }
      frame "PPSU_DC_ON" {
        n202 = call "ATF_PPSU ON.vi"("error in"=w332) -> ("Fehler"=w333:errorcluster)  [unwired: 26 in]
        n203 = Merge Errors(w333) -> (w334:errorcluster)
      }
      frame "PPSU_DC_OFF" {
        n204 = call "ATF_PPSU OFF.vi"("Error in"=w335) -> ("Fehler"=w336:errorcluster)  [unwired: 26 in]
        n205 = Merge Errors(w336) -> (w337:errorcluster)
      }
      frame "Control_Valve" {
        n206 = Variant To Data(error in=w342, type=0.0, Variant=w339) -> (data=w338:dbl, error out=w341:errorcluster)
        n207 = global write "ATF1_ACQ.vi" "AO_Array"(w338) -> ()
        n208 = Merge Errors(w341) -> (w343:errorcluster)
      }
      frame "PPSU_Ack_Alarm" {
        n209 = call "ACK Alarm.vi"("error in"=w345) -> ("Fehler"=w344:errorcluster)  [unwired: 26 in]
        n210 = Merge Errors(w344) -> (w346:errorcluster)
      }
      frame "PPSU_MS_Init" {
        n211 = call "ATF_Init_MS.vi"("error in"=w348) -> ("Fehler"=w347:errorcluster)  [unwired: 26 in]
        n212 = Merge Errors(w347) -> (w349:errorcluster)
      }
      frame "PPSU Enable" {
        n213 = flat-sequence {
          tunnel: w353 -> [w355]
          tunnel: [w355] -> w351
          tunnel: w351 -> [w356]
          tunnel: [w356] -> w350
          tunnel: [w363] -> w352
          tunnel: w350 -> [w363]
          frame #0 {
            n214 = call "ATF_Ex_master-slave_ELR_PSI_PSE_PSB.vi"() -> ()  [unwired: 1 in]
            n215 = global write "Main_global.vi" "PPSU Enable"(TRUE ("UI Exit")) -> ()
          }
          frame #1 {
            n216 = disable-structure shown="Disabled" {
              frame Disabled {
                n217 = global read "ATF1_ACQ.vi" "set Voltage"() -> (w361:dbl)
                n218 = global read "ATF1_ACQ.vi" "set Current"() -> (w359:dbl)
                n219 = global read "ATF1_ACQ.vi" "set Power"() -> (w357:dbl)
                n220 = global read "ATF1_ACQ.vi" "OPP(W)"() -> (w358:dbl)
                n221 = global read "ATF1_ACQ.vi" "OCP(A)"() -> (w360:dbl)
                n222 = global read "ATF1_ACQ.vi" "OVP(V)"() -> (w362:dbl)
                n223 = call "ATF_PPSU control1.vi"("OVP"=w362, "set Voltage"=w361, "OCP"=w360, "set current"=w359, "OPP"=w358, "set Power"=w357) -> ()  [unwired: 20 in, 2 out]
              }
              frame Enabled {
              }
            }
          }
          frame #2 {
            n224 = disable-structure shown="Disabled" {
              frame Disabled {
                n225 = call "ATF1_File and Folder Info.vi"() -> ("Path Cluster 3"=w365:T6)  [unwired: 10 in, 1 out]
                n226 = Unbundle By Name(w365) -> ("Loading Vi path"=w364:path)
                n227 = call "call by reference.vi"("vi path"=w364) -> ()  [unwired: 10 in]
              }
              frame Enabled {
              }
            }
          }
        }
      }
      frame "Drive_Switching_Frequency" {
        n228 = Variant To Data(error in=w371, type=0.0 ("Drive_Switching Freq."), Variant=w370) -> (data=w369:dbl, error out=w367:errorcluster)
        n229 = global read "ATF1_ACQ.vi" "Drive_Enable"() -> (w366:bool)
        n230 = case shown="True" w366 {
          tunnel: w369 -> [_ w380]
          tunnel: [w374 w378] -> w368
          tunnel: w367 -> [w374 w377]
          frame False {
          }
          frame True {
            n231 = global read "ATF1_ACQ.vi" "connection ID"() -> (w375:refnum<k5>)
            n232 = call "ATF1_Drive_messsage.vi"("Numeric"=18, "Switching Freq."=w380) -> ("String"=w376:string)  [unwired: 9 in]
            n233 = TCP Write(connection ID=w375, data in=w376, error in (no error)=w377) -> (error out=w378:errorcluster)  [unwired: 1 in, 2 out]
          }
        }
        n234 = Merge Errors(w368) -> (w373:errorcluster)
      }
      frame "Drive_Speed" {
        n235 = Variant To Data(error in=w387, type=0.0 ("Speed (RPM)"), Variant=w386) -> (data=w381:dbl, error out=w383:errorcluster)
        n236 = global read "ATF1_ACQ.vi" "Drive_Enable"() -> (w384:bool)
        n237 = case shown="True" w384 {
          tunnel: w381 -> [_ w394]
          tunnel: w383 -> [w389 w392]
          tunnel: [w389 w391] -> w382
          frame False {
          }
          frame True {
            n238 = global read "ATF1_ACQ.vi" "connection ID"() -> (w390:refnum<k5>)
            n239 = call "ATF1_Drive_messsage.vi"("Numeric"=21, "Switching Freq."=w394) -> ("String"=w393:string)  [unwired: 9 in]
            n240 = TCP Write(connection ID=w390, data in=w393, error in (no error)=w392) -> (error out=w391:errorcluster)  [unwired: 1 in, 2 out]
          }
        }
        n241 = global write "ATF1_ACQ.vi" "Drive set_RPM"(w381) -> ()
        n242 = Merge Errors(w382) -> (w388:errorcluster)
      }
      frame "Drive _Ramp _UP_Time" {
        n243 = global read "ATF1_ACQ.vi" "Drive_Enable"() -> (w396:bool)
        n244 = Variant To Data(error in=w402, type=0.0, Variant=w400) -> (data=w399:dbl, error out=w397:errorcluster)
        n245 = case shown="True" w396 {
          tunnel: w399 -> [_ w409]
          tunnel: [w404 w408] -> w398
          tunnel: w397 -> [w404 w407]
          frame False {
          }
          frame True {
            n246 = call "ATF1_Drive_messsage.vi"("Numeric"=19, "Switching Freq."=w409) -> ("String"=w406:string)  [unwired: 9 in]
            n247 = global read "ATF1_ACQ.vi" "connection ID"() -> (w405:refnum<k5>)
            n248 = TCP Write(connection ID=w405, data in=w406, error in (no error)=w407) -> (error out=w408:errorcluster)  [unwired: 1 in, 2 out]
          }
        }
        n249 = Merge Errors(w398) -> (w403:errorcluster)
      }
      frame "Drive_Ramp_Down_Time" {
        n250 = Variant To Data(error in=w416, type=0.0, Variant=w415) -> (data=w414:dbl, error out=w413:errorcluster)
        n251 = global read "ATF1_ACQ.vi" "Drive_Enable"() -> (w411:bool)
        n252 = case shown="True" w411 {
          tunnel: w414 -> [_ w424]
          tunnel: w413 -> [w419 w421]
          tunnel: [w419 w422] -> w412
          frame False {
          }
          frame True {
            n253 = call "ATF1_Drive_messsage.vi"("Numeric"=20, "Switching Freq."=w424) -> ("String"=w423:string)  [unwired: 9 in]
            n254 = global read "ATF1_ACQ.vi" "connection ID"() -> (w420:refnum<k5>)
            n255 = TCP Write(connection ID=w420, data in=w423, error in (no error)=w421) -> (error out=w422:errorcluster)  [unwired: 1 in, 2 out]
          }
        }
        n256 = Merge Errors(w412) -> (w418:errorcluster)
      }
      frame "Drive_Motor_ON" {
        n257 = global read "ATF1_ACQ.vi" "Drive_Enable"() -> (w428:bool)
        n258 = global read "ATF1_ACQ.vi" "connection ID"() -> (w426:refnum<k5>)
        n259 = case shown="True" w428 {
          tunnel: [w431 w436] -> w427
          tunnel: w429 -> [w431 w435]
          tunnel: w426 -> [_ w432]
          frame False {
          }
          frame True {
            n260 = call "ATF1_Drive_messsage.vi"("Numeric"=17, "Switching Freq."=1.0) -> ("String"=w433:string)  [unwired: 9 in]
            n261 = TCP Write(connection ID=w432, data in=w433, error in (no error)=w435) -> (error out=w436:errorcluster)  [unwired: 1 in, 2 out]
          }
        }
        n262 = Merge Errors(w427) -> (w430:errorcluster)
      }
      frame "Drive_Exit" {
        n263 = global write "ATF1_ACQ.vi" "Drive_Exit"(TRUE ("Drive_Exit")) -> ()
        n264 = global read "ATF1_ACQ.vi" "connection ID"() -> (w438:refnum<k5>)
        n265 = global write "ATF1_ACQ.vi" "Drive_Enable"(FALSE ("Drive Connected?")) -> ()
        n266 = TCP Close Connection(connection ID=w438, error in (no error)=w439) -> (error out=w440:errorcluster)  [unwired: 1 in, 1 out]
        n267 = Merge Errors(w440) -> (w443:errorcluster)
      }
      frame "Drive_Enable" {
        n268 = Variant To Data(error in=w449, type=TRUE, Variant=w446) -> (data=w445:bool, error out=w448:errorcluster)
        n269 = flat-sequence {
          frame #0 {
            n270 = global read "ATF1_ACQ.vi" "TCP port"() -> (w450:dbl)
          }
          frame #1 {
            n271 = disable-structure shown="Disabled" {
              frame Disabled {
                n272 = call "ATF1_File and Folder Info.vi"() -> ("Path Cluster 3"=w451:T6)  [unwired: 10 in, 1 out]
                n273 = Unbundle By Name(w451) -> ("Loading Vi path D"=w452:path)
                n274 = call "call by reference.vi"("vi path"=w452) -> ()  [unwired: 10 in]
              }
              frame Enabled {
              }
            }
          }
        }
        n275 = global write "ATF1_ACQ.vi" "Drive_Enable"(w445) -> ()
        n276 = global write "ATF1_ACQ.vi" "Drive_Exit"(FALSE ("Drive_Exit")) -> ()
      }
      frame "Drive_Motor_OFF" {
        n277 = call "ATF1_Drive_messsage.vi"("Numeric"=17, "Switching Freq."=0.0) -> ("String"=w456:string)  [unwired: 9 in]
        n278 = global read "ATF1_ACQ.vi" "connection ID"() -> (w453:refnum<k5>)
        n279 = TCP Write(connection ID=w453, data in=w456, error in (no error)=w454) -> (error out=w455:errorcluster)  [unwired: 1 in, 2 out]
        n280 = Merge Errors(w455) -> (w459:errorcluster)
      }
      frame "Signal_List" {
        n281 = flat-sequence {
          tunnel: w461 -> [w463]
          tunnel: [w463] -> w460
          frame #0 {
            n282 = call "signal list.vi"() -> ()  [unwired: 12 in]
          }
        }
        n283 = Merge Errors(w460) -> (w462:errorcluster)
      }
      frame "VFD_OFF" {
        n284 = Variant To Data(error in=w466, type=0.0, Variant=w464) -> (data=w468:dbl, error out=w465:errorcluster)
        n285 = global write "ATF1_ACQ.vi" "VFD_OFF"(w468) -> ()
        n286 = Merge Errors(w465) -> (w469:errorcluster)
      }
      frame "VFD_Exit" {
        n287 = Merge Errors(w470) -> (w471:errorcluster)
      }
      frame "Start Datalog" {
        w478 = T2."Enabled" ("Disabled")
        w481 = T2."Disabled and Grayed Out" ("Disabled")
        n288 = Variant To Data(error in=w476, type=bool[] [], Variant=w486) -> (data=w484:bool[], error out=w480:errorcluster)
        n289 = Index Array(array=w484) -> (element #1=w483:bool, element #2=w482:bool)  [unwired: 2 in]
        n290 = global write "Main_global.vi" "Start Datalog"(w483) -> ()
        n291 = global write "Main_global.vi" "Stop Datalog"(w482) -> ()
        n292 = call "ATF_Enqueue Message.vi"("error in (no error)"=w476, "Message"="Start", "Message Queue"=w477) -> ("error out"=w474:errorcluster)  [unwired: 7 in, 1 out]
        n293 = global read "Main_global.vi" "datalog prefix"() -> (w472:string)
        n294 = Merge Errors(w474) -> (w475:errorcluster, w479:errorcluster)
      }
      frame "Rename_Datalog" {
        w493 = T2."Enabled" ("Disabled")
        w495 = T2."Enabled" ("Disabled")
        n295 = global read "Main_global.vi" "Start Datalog"() -> (w487:bool)
        n296 = case shown="False" w487 {
          tunnel: [w496 w503] -> w491
          tunnel: w489 -> [w496 w500]
          tunnel: w488 -> [_ w499]
          frame False {
          }
          frame True {
            n297 = call "ATF_Enqueue Message.vi"("error in (no error)"=w500, "Message"="Stop", "Message Queue"=w499) -> ("error out"=w501:errorcluster, "dup Message Queue"=w498:refnum<queue>)  [unwired: 7 in]
            n298 = call "ATF_Enqueue Message.vi"("error in (no error)"=w501, "Message"="Start", "Message Queue"=w498) -> ("error out"=w503:errorcluster)  [unwired: 7 in, 1 out]
          }
        }
        n299 = local read item#-1() -> (w490)
        n300 = global write "Main_global.vi" "datalog prefix"(w490) -> ()
        n301 = Merge Errors(w491) -> (w492:errorcluster, w494:errorcluster)
      }
      frame "Stop Datalog" {
        w509 = T2."Disabled and Grayed Out" ("Disabled")
        w510 = T2."Enabled" ("Disabled")
        n302 = Variant To Data(error in=w508, type=bool[] [], Variant=w517) -> (data=w515:bool[], error out=w512:errorcluster)
        n303 = Index Array(array=w515) -> (element #1=w514:bool, element #2=w513:bool)  [unwired: 2 in]
        n304 = global write "Main_global.vi" "Start Datalog"(w514) -> ()
        n305 = global write "Main_global.vi" "Stop Datalog"(w513) -> ()
        n306 = call "ATF_Enqueue Message.vi"("error in (no error)"=w508, "Message"="Stop", "Message Queue"=w507) -> ("error out"=w505:errorcluster)  [unwired: 7 in, 1 out]
        n307 = Merge Errors(w505) -> (w506:errorcluster, w511:errorcluster)
      }
      frame "RT Connect" {
        n308 = call "ATF_NS_Storage.vi"("error in (no error)"=w523, "Message Queue"=w524) -> ("error out"=w526:errorcluster, "Connected?"=w525:bool, "Target IP Address:"=w528:string)  [unwired: 7 in]
        n309 = call "ATF_Enqueue Message.vi"("error in (no error)"=w523, "Message"="Write DO_P ", "Message Queue"=w524) -> ("error out"=w521:errorcluster, "dup Message Queue"=w519:refnum<queue>)  [unwired: 7 in]
        n310 = call "ATF_Enqueue Message.vi"("error in (no error)"=w521, "Message"="Write DO_S ", "Message Queue"=w519) -> ("error out"=w520:errorcluster)  [unwired: 7 in, 1 out]
        n311 = Merge Errors(w520, w526) -> (w527:errorcluster)
      }
      frame "Write DO_P" {
        w530 = FALSE ("element")
        n312 = global read "ATF1_ACQ.vi" "Gate Driver Reset"() -> (w529:bool)
        n313 = Build Array("F EPV 1004", "F EPV 1008", "N EPV 1091", "NC EPV 1217", w529, w530, w530) -> (w532:bool[])
        n314 = global write "ATF1_ACQ.vi" "DO Array_P"(w532) -> ()
      }
      frame "Update DO_S" {
        n315 = global read "ATF1_ACQ.vi" "DO Array_S"() -> (w537:bool[])
        n316 = global read "Main_global.vi" "DO_Index_T2"() -> (w543:i32[])
        n317 = for {
          tunnel: w537 -> [w546]
          tunnel: w543 -> [w545] mode=indexing
          tunnel: [w544] -> w542 mode=indexing
          n318 = Index Array(array=w546, index=w545) -> (element=w544:bool)
        }
        n319 = Index Array(array=w542) -> (element #1=w541:bool, element #2=w540:bool, element #3=w539:bool, element #4=w538:bool)  [unwired: 4 in]
        n320 = local write "NO EPV 1102"(w541) -> ()
        n321 = local write "NC EPV 1211"(w540) -> ()
        n322 = local write "NC EPV 1214"(w539) -> ()
        n323 = local write "NO EPV 1207"(w538) -> ()
      }
      frame "Update DO_P" {
        n324 = global read "ATF1_ACQ.vi" "DO Array_P"() -> (w547:bool[])
        n325 = global read "Main_global.vi" "DO_Index_T1"() -> (w553:i32[])
        n326 = for {
          tunnel: w547 -> [w556]
          tunnel: w553 -> [w555] mode=indexing
          tunnel: [w554] -> w552 mode=indexing
          n327 = Index Array(array=w556, index=w555) -> (element=w554:bool)
        }
        n328 = Index Array(array=w552) -> (element #1=w551:bool, element #2=w550:bool, element #3=w549:bool, element #4=w548:bool)  [unwired: 4 in]
        n329 = local write "F EPV 1004"(w551) -> ()
        n330 = local write "F EPV 1008"(w550) -> ()
        n331 = local write "N EPV 1091"(w549) -> ()
        n332 = local write "NC EPV 1217"(w548) -> ()
        n333 = disable-structure shown="Disabled" {
          frame Disabled {
            n334 = local read item#-1() -> ()  [unwired: 1 in]
            n335 = local read item#-1() -> ()  [unwired: 1 in]
            n336 = local read item#-1() -> ()  [unwired: 1 in]
          }
          frame Enabled {
          }
        }
      }
      frame "DAQ_Configuration" {
        n337 = flat-sequence {
          frame #0 {
            w565 = T8 0 items=["no dialog", "OK message", "continue or stop message", "OK message + warnings", "continue/stop + warnings"] ("type of dialog (OK msg:1)")
            n338 = call "ATF1_File and Folder Info.vi"() -> ("Path Cluster 3"=w561:T6)  [unwired: 10 in, 1 out]
            n339 = Unbundle By Name(w561) -> ("Sub VI's  Folder Path"=w562:path)
            n340 = Build Path(base path=w562, name or relative path=path "Hardware_Configuration.vi") -> (appended path=w563:path)
            n341 = Open VI Reference(vi path=w563) -> (vi reference=w574:refnum<vi>, error out=w573:errorcluster)  [unwired: 5 in]
            n342 = invoke class="VI" method="FP.Open"(reference=w574, error in=w573, "Activate"=TRUE ("Activate?"), "State"=T5."Standard") -> (reference out=w572:refnum<vi>, error out=w571:errorcluster)  [unwired: 1 in, 3 out]
            n343 = invoke class="VI" method="Run VI"(reference=w572, error in=w571, "Wait until done"=TRUE ("Wait Until Done"), "Auto Dispose Ref"=FALSE ("Auto Dispose Reference")) -> (reference out=w560:refnum<vi>, error out=w558:errorcluster)  [unwired: 1 in, 3 out]
            n344 = invoke class="VI" method="FP.Close"(reference=w560, error in=w558) -> (reference out=w559:refnum<vi>, error out=w557:errorcluster)  [unwired: 1 in, 1 out]
            n345 = Close Reference(reference=w559, error in (no error)=w557) -> (error out=w566:errorcluster)
            n346 = call <vilib>:"Simple Error Handler.vi"("type of dialog (OK msg:1)"=w565, "error in (no error)"=w566) -> ()  [unwired: 3 in, 5 out]
          }
        }
      }
      frame "Edit IP" {
        w575 = T2."Enabled" ("Disabled")
      }
      frame "Write DO_S" {
        n347 = local read item#-1() -> (w583)
        n348 = Build Array("NC EPV 1211", "NO EPV 1102", "NC EPV 1214", "NO EPV 1207", "AC Button") -> (w584:bool[])
        n349 = case shown="True" w583 {
          tunnel: [w588 w594] -> w586
          tunnel: w584 -> [_ w593]
          tunnel: w585 -> [_ w592]
          tunnel: w587 -> [w588 w590]
          frame False {
          }
          frame True {
            n350 = global read "ATF1_NS_globals.vi" "UI Command Stream_S"() -> (w589:refnum<k21>)
            n351 = Bundle(w592, w593) -> (w591:cluster{string, bool[]})  [unwired: 1 in]
            n352 = shared-variable-write(w589, w590, w591) -> (w594:errorcluster)  [unwired: 1 in, 2 out]
          }
        }
      }
      frame "Indexing" {
        n353 = flat-sequence {
          tunnel: w596 -> [w598]
          tunnel: [w598] -> w595
          frame #0 {
            n354 = call "ATF1_Indexing.vi"() -> ()  [unwired: 12 in]
          }
        }
        n355 = Merge Errors(w595) -> (w597:errorcluster)
      }
      frame "Update_HW_File_List" {
        n356 = call "ATF1_File and Folder Info.vi"() -> ("Path Cluster 3"=w601:T6)  [unwired: 10 in, 1 out]
        n357 = Unbundle By Name(w601) -> ("HW Configaration  Folder Path"=w600:path)
        n358 = List Folder(path=w600) -> (filenames=w599:string[])  [unwired: 3 in, 3 out]
      }
    }
    n359 = global read "Main_global.vi" "UI Exit"() -> (w188:bool)
    n360 = call <vilib>:"Clear Errors.vi"("error in (no error)"=w190) -> ("error out"=w189:errorcluster)  [unwired: 5 in, 1 out]
  }
  n361 = while {
    tunnel: w14 -> [w627]
    tunnel: w16 -> [w626]
    stop <- w625 stop-if-true
    # "ATF Storage Area Sensor Update"
    n362 = Wait on Notification(notifier=w627, error in (no error)=w626) -> (notification=w611:T1, error out=w625:errorcluster)  [unwired: 2 in, 2 out]
    n363 = Unbundle By Name(w611) -> ("AI Data"=w622:waveform(dbl)[], "DI Data"=w605:digitalwaveform[])
    n364 = for {
      tunnel: [w641] -> _ mode=indexing
      tunnel: w605 -> [w640] mode=indexing
      n365 = call-poly <vilib>:"Digital to Boolean Array.vi"("digital waveform"=w640) -> ("boolean array"=w642:bool[][])  [unwired: 9 in, 1 out]
      n366 = Or Array Elements(Boolean array=w642) -> (logical OR=w641:bool)
    }
    n367 = for {
      tunnel: w622 -> [w647] mode=indexing
      tunnel: [w649] -> w623 mode=indexing
      n368 = Unbundle By Name(w647) -> ("Y"=w646:dbl[])
      n369 = Index Array(array=w646, index=0) -> (element=w649:dbl)
    }
    n370 = global read "Main_global.vi" "AI_Index_T2"() -> (w624:i32[])
    n371 = for {
      tunnel: w605 -> [w631] mode=indexing
      tunnel: [w628] -> w603 mode=indexing
      n372 = Unbundle By Name(w631) -> ("Y"=w630:digitaldata)
      n373 = Unbundle By Name(w630) -> ("data"=w629:u8[][])
      n374 = for {
        tunnel: w629 -> [w633] mode=indexing
        tunnel: [w632] -> w628
        n375 = for {
          tunnel: w633 -> [w639] mode=indexing
          tunnel: [w634] -> w632
          n376 = call <vilib>:"Butterworth Filter PtByPt.vi"("order"=4, "filter type"=Filter_Passband_Type."Lowpass", "low cutoff freq: fl"=10.0, "x"=w639) -> ("Filtered x"=w635:dbl)  [unwired: 5 in, 1 out]
          n377 = Number To Boolean Array(number=w635) -> (Boolean array=w634:bool[])
        }
      }
    }
    n378 = for {
      tunnel: w623 -> [w645]
      tunnel: [w644] -> w621 mode=indexing
      tunnel: w624 -> [w643] mode=indexing
      n379 = Index Array(array=w645, index=w643) -> (element=w644:dbl)
    }
    n380 = Index Array(array=w621) -> (element #1=w610:dbl, element #2=w609:dbl, element #3=w608:dbl, element #4=w607:dbl, element #5=w606:dbl)  [unwired: 5 in]
    n381 = Compound Arithmetic op=MULTIPLY(10.0 ("value"), 998.0 ("value"), 9.81 ("value")) -> (w620:dbl)
    n382 = Divide(x=w606, y=w620) -> (x/y=→"WTT_LS":dbl)
    n383 = Index Array(array=w603, index (col)=0 ("disabled index (col)")) -> (element=w602:bool[])  [unwired: 1 in]
    n384 = Index Array(array=w602) -> (element #1=→"NO EPV 1102 HSS":bool, element #2=→"NC EPV 1211 HSS":bool, element #3=→"NC EPV 1214 HSS":bool, element #4=→"NO EPV 1207 HSS":bool)  [unwired: 4 in]
  }
  n385 = Unregister For Events(event registration refnum=w10, error in=w11) -> (error out=w9:errorcluster)
  n386 = Release Queue(queue=w23, error in (no error)=w22) -> (error out=w21:errorcluster)  [unwired: 1 in, 2 out]
  n387 = Merge Errors(w9, w21, w20, w18, w5) -> (w8:errorcluster)
  n388 = call "Destroy User Event - Stop.vi"("error in (no error)"=w8, "User Event - Stop"=w6) -> ("error out"=→"error out":errorcluster)  [unwired: 9 in]
  n389 = disable-structure shown="Enabled" {
    frame Disabled {
    }
    frame Enabled {
    }
  }
  n390 = disable-structure shown="Disabled" {
    frame Disabled {
      # "buttons and control"
      # "health status"
    }
    frame Enabled {
    }
  }
  n391 = disable-structure shown="Disabled" {
    frame Disabled {
      n392 = global read "Main_global.vi" "Stop DAQ"() -> ()  [unwired: 1 out]
    }
    frame Enabled {
    }
  }
  n393 = disable-structure shown="Disabled" {
    frame Disabled {
      n394 = global read "Main_global.vi" "Acc_Data_P"() -> ()  [unwired: 1 in]
      n395 = global read "Main_global.vi" "TC_Data_P"() -> ()  [unwired: 1 in]
      n396 = global read "Main_global.vi" "Voltage_Data_P"() -> ()  [unwired: 1 in]
    }
    frame Enabled {
    }
  }
